vi "Write window position to ini file & close.vi"(7 "Window Name":string, 8 "Front Panel.WinBounds":T2, 9 "FP.State":T1(ring)=enum."Standard", 10 "Disable closing":bool, 11 "VI in":refnum<vi>) -> ()   [LabVIEW 2017]
uses:
  <vilib>/Utility/miscctls.llb/LVRectTypeDef.ctl
  Typedefs/Which path.ctl
  <vilib>/Utility/config.llb/Write Key (String).vi
  <vilib>/Utility/config.llb/NI_LVConfig.lvlib
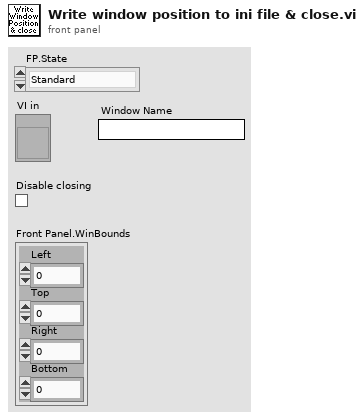
[diagram p1: front panel]
types:
  T1 = enum32{"Invalid", "Standard", "Closed", "Hidden", "Minimized", "Maximized"}
  T2 = typedef "LVRectTypeDef.ctl" = cluster{"Left":i16, "Top":i16, "Right":i16, "Bottom":i16}
  T3 = typedef "Which path.ctl" = enum16{"Configuration Files", "Calibration Files", "Images", "Setup.ini", "Loaded User profile.ini", "User's-Previous session.ini", "New user profile.ini", "Selected User profile.ini", "User profiles folder", "Power meter scaling.txt", "FOV Cal.ini"}
  T4 = typedef "NI_LVConfig.lvlib/Config Data RefNum.ctl" = refnum<k1>
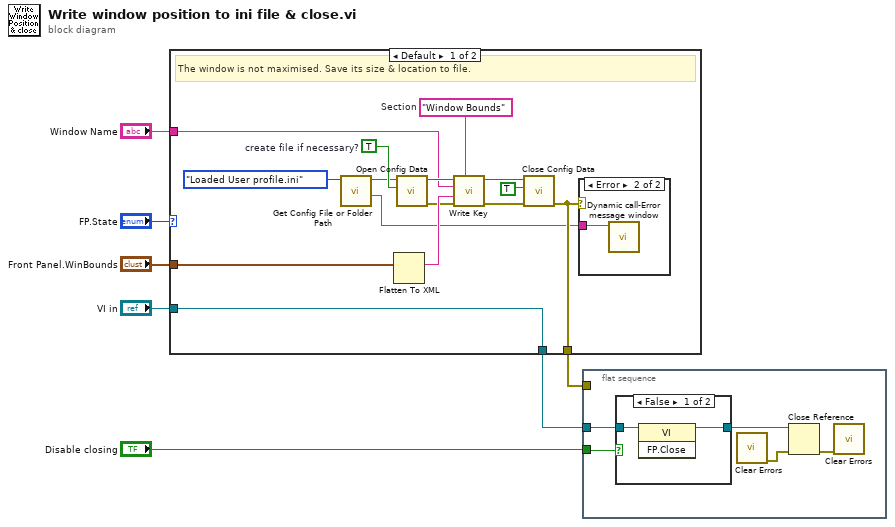
[diagram p0: block diagram]
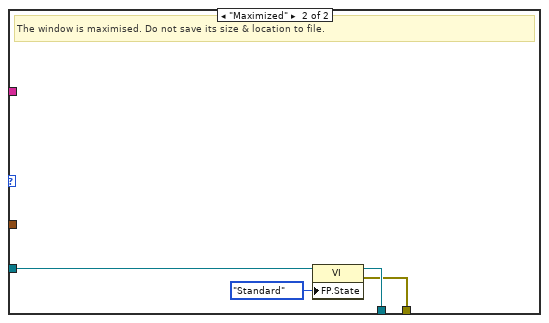
[diagram p3: hidden frame]
diagram:
  n1 = case shown="Default" "FP.State" {
    tunnel: "Front Panel.WinBounds" -> [w22 _]
    tunnel: "Window Name" -> [w13 _]
    tunnel: [w12 w24] -> w4
    tunnel: "VI in" -> [w11 w25]
    tunnel: [w11 w27] -> w1
    frame Default {
      w16 = "Window Bounds"  # Section
      w15 = TRUE  # create file if necessary?
      # "The window is not maximised. Save its size & location to file."
      n2 = call "Get Config File or Folder Path.vi"("Which file or folder?"=Which_path."Loaded User profile.ini" ("Which path?")) -> ("File/Folder name string"=w8:string, "File Path"=w9:path)  [unwired: 8 in, 1 out]
      n3 = Flatten To XML(anything=w22) -> (xml string=w21:string)
      n4 = call <vilib>:"Open Config Data.vi"("create file if necessary (T)"=w15, "configuration file path"=w9) -> ("error out"=w18:errorcluster, "refnum"=w17:T4)  [unwired: 7 in, 1 out]
      n5 = call-poly <vilib>:"Write Key.vi"("section"=w16, "error in (no error)"=w18, "value"=w21, "key"=w13, "refnum"=w17) -> ("error out"=w20:errorcluster, "refnum out"=w19:T4)  [unwired: 4 in, 1 out]
      n6 = call <vilib>:"Close Config Data.vi"("error in (no error)"=w20, "write file if changed (T)"=TRUE ("write configuration file? (F)"), "refnum"=w19) -> ("error out"=w12:errorcluster)  [unwired: 7 in, 1 out]
      n7 = case shown="Error" w12 {
        tunnel: w8 -> [_ w23]
        frame No Error {
        }
        frame Error {
          n8 = call "Dynamic call-Error message window.vi"("Error Message"=w23) -> ()  [unwired: 10 in, 1 out]
        }
      }
    }
    frame "Maximized" {
      # "The window is maximised. Do not save its size & location to file."
      n9 = property class="VI"(reference=w25, "FP.State"=T1."Standard" ("Front Panel Window:State")) -> (reference out=w27:refnum<vi>, error out=w24:errorcluster)  [unwired: 1 in]
    }
  }
  n10 = flat-sequence {
    tunnel: w1 -> [w30]
    tunnel: "Disable closing" -> [w28]
    tunnel: w4 -> [_]
    frame #0 {
      n11 = case shown="False" w28 {
        tunnel: w30 -> [w34 w35]
        tunnel: [w33 w35] -> w29
        frame False {
          n12 = invoke class="VI" method="FP.Close"(reference=w34) -> (reference out=w33:refnum<vi>)  [unwired: 2 in, 2 out]
        }
        frame True {
        }
      }
      n13 = call <vilib>:"Clear Errors.vi"() -> ("error out"=w32:errorcluster)  [unwired: 6 in, 1 out]
      n14 = Close Reference(reference=w29, error in (no error)=w32) -> (error out=w31:errorcluster)
      n15 = call <vilib>:"Clear Errors.vi"("error in (no error)"=w31) -> ()  [unwired: 5 in, 2 out]
    }
  }
